vi "c_n__v1.vi"(0 "配列":ext[][](array[numeric]), 6 "D":ext, 8 "R":ext, 10 "n":ext) -> (14 "c[n]":ext format="%#.6g")   [LabVIEW 2020]
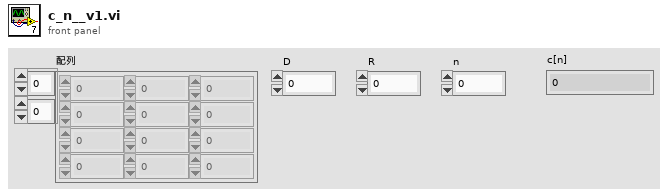
[diagram p1: front panel]
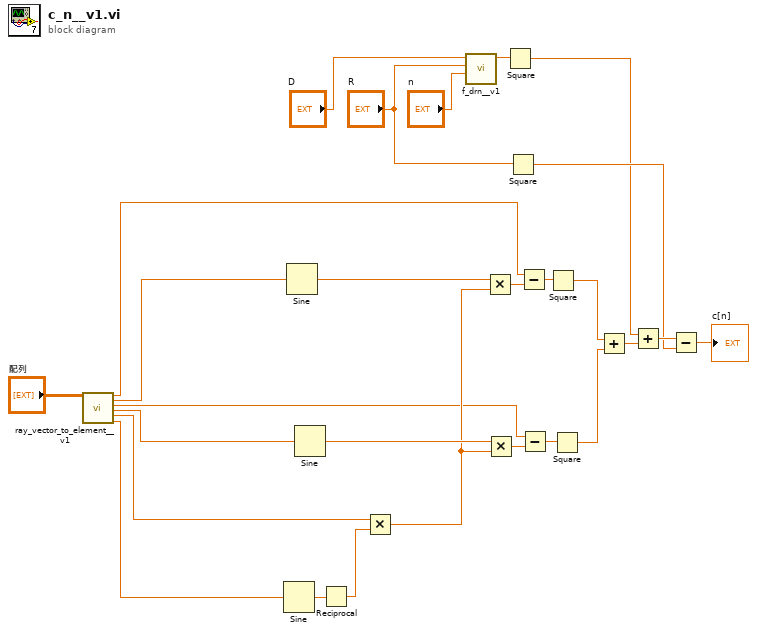
[diagram p0: block diagram]
diagram:
  n1 = call "ray_vector_to_element__v1.vi"("光線ベクトル"="配列") -> ("x"=w6:ext, "α"=w5:ext, "y"=w4:ext, "β"=w3:ext, "z"=w2:ext, "γ"=w1:ext)  [unwired: 13 in]
  n2 = Sine(x=w1) -> (sin(x)=w27:ext)
  n3 = Sine(x=w5) -> (sin(x)=w10:ext)
  n4 = Sine(x=w3) -> (sin(x)=w12:ext)
  n5 = Reciprocal(x=w27) -> (1/x=w13:ext)
  n6 = Multiply(x=w2, y=w13) -> (x*y=w11:ext)
  n7 = call "f_drn__v1.vi"("n"="n", "R"="R", "D"="D") -> ("出力結果"=w18:ext)  [unwired: 8 in]
  n8 = Multiply(x=w10, y=w11) -> (x*y=w24:ext)
  n9 = Multiply(x=w12, y=w11) -> (x*y=w23:ext)
  n10 = Square(x=w18) -> (x^2=w8:ext)
  n11 = Square(x="R") -> (x^2=w15:ext)
  n12 = Subtract(x=w6, y=w24) -> (x-y=w22:ext)
  n13 = Subtract(x=w4, y=w23) -> (x-y=w21:ext)
  n14 = Square(x=w22) -> (x^2=w20:ext)
  n15 = Square(x=w21) -> (x^2=w19:ext)
  n16 = Add(x=w20, y=w19) -> (x+y=w9:ext)
  n17 = Add(x=w8, y=w9) -> (x+y=w16:ext)
  n18 = Subtract(x=w16, y=w15) -> (x-y=→"c[n]":ext)
